vi "Logging Infor.vi"(8 "error in":errorcluster, 10 "error in (no error)":errorcluster, 11 "Class":refnum<class>) -> (0 "error out":errorcluster)   [LabVIEW 2020, in "MMVVM Framework.lvlib" / "MVVM Abstruct Model.lvlib" / "MVVM Abstruct Model.lvclass"]
uses:
  MVVM Framework/MVVM Abstruct Model/MVVM Abstruct Model/MVVM Abstruct Model.lvclass
  <vilib>/Utility/file.llb/Write Delimited Spreadsheet (string).vi
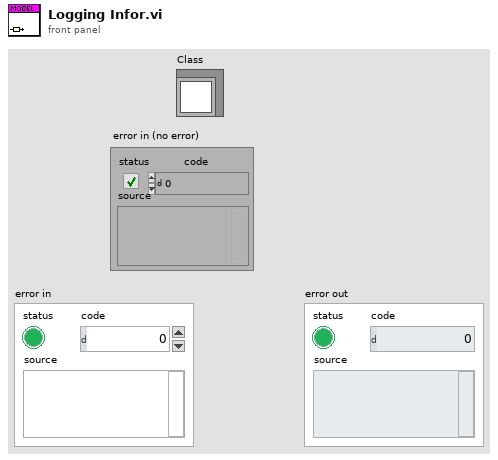
[diagram p1: front panel]
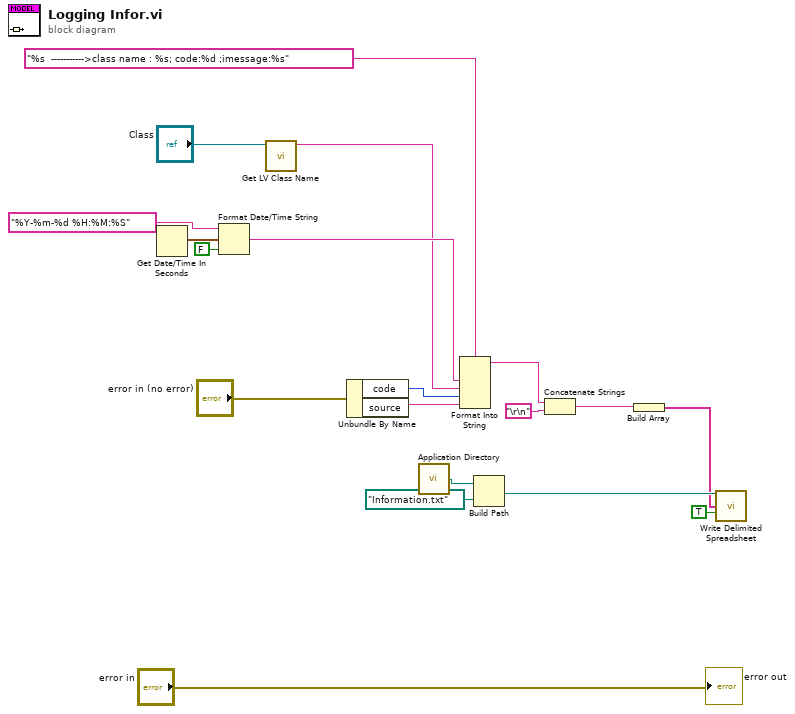
[diagram p0: block diagram]
diagram:
  n1 = Get Date/Time In Seconds() -> (seconds since 1Jan1904=w13:timestamp)
  n2 = Format Date/Time String(time format string (%c)="%Y-%m-%d %H:%M:%S", seconds (now)=w13, UTC format=FALSE) -> (date/time string=w10:string)
  n3 = call <vilib>:"Get LV Class Name.vi"("object"="Class") -> ("class name"=w9:string)  [unwired: 9 in, 1 out]
  n4 = Unbundle By Name("error in (no error)") -> ("code"=w8:i32, "source"=w16:string)
  n5 = call <vilib>:"Application Directory.vi"() -> ("Application Directory"=w15:path)
  n6 = Format Into String(format string="%s  ----------->class name : %s; code:%d ;imessage:%s", w10, w9, w8, w16) -> (resulting string=w7:string)  [unwired: 2 in, 1 out]
  n7 = Build Path(base path=w15, name or relative path=path "Information.txt") -> (appended path=w6:path)
  n8 = Concatenate Strings(w7, "\r\n") -> (w4:string)
  n9 = Build Array(w4) -> (w3:string[])
  n10 = call-poly <vilib>:"Write Delimited Spreadsheet.vi"("file path (dialog if empty)"=w6, "1D data"=w3, "append to file? (new file:F)"=TRUE) -> ()  [unwired: 11 in, 2 out]
  "error out" <- "error in"
